vi "BuildFilterInput32.vi"(10 "Q in":fxp<+/-,32,14>, 11 "I in":fxp<+/-,32,14>) -> (3 "Filter input":fxp<+,64,64>)   [LabVIEW 2018]
uses:
  <vilib>/rvi/FXPMathLib/FxpInterpret/XNode/nifxpmath_Interpret.xnode
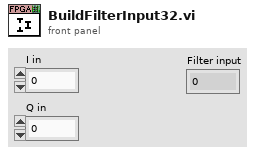
[diagram p1: front panel]
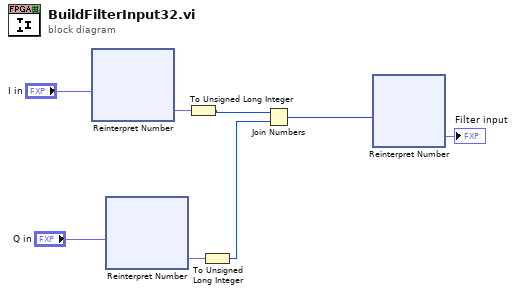
[diagram p0: block diagram]
diagram:
  n1 = xnode "Reinterpret Number"("x"="I in") -> ("y"=w7:fxp<+,32,32>)
  n2 = xnode "Reinterpret Number"("x"="Q in") -> ("y"=w4:fxp<+,32,32>)
  n3 = To Unsigned Long Integer(number=w7) -> (unsigned 32bit integer=w5:u32)
  n4 = To Unsigned Long Integer(number=w4) -> (unsigned 32bit integer=w2:u32)
  n5 = Join Numbers(hi=w5, lo=w2) -> ((hi.lo)=w8:u64)
  n6 = xnode "Reinterpret Number"("x"=w8) -> ("y"=→"Filter input":fxp<+,64,64>)
